vi "parse.issues.vi"(7 "series body":string, 8 "error in (no error)":errorcluster, 11 "ComicVine_class in":refnum<class "series_class.lvclass">) -> (0 "error out":errorcluster, 3 "ComicVine_class out":refnum<class "series_class.lvclass">)   [LabVIEW 2024, in "series_class.lvclass"]
uses:
  series_class.lvclass
  series_class.lvclass/series_class.ctl
  issue_class/issue_class.lvclass
  comic_class/comic_class.lvclass
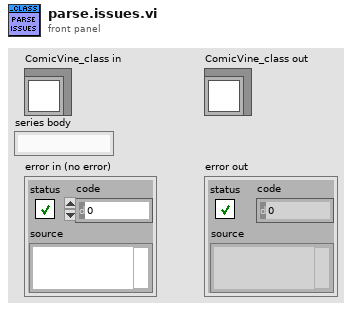
[diagram p1: front panel]
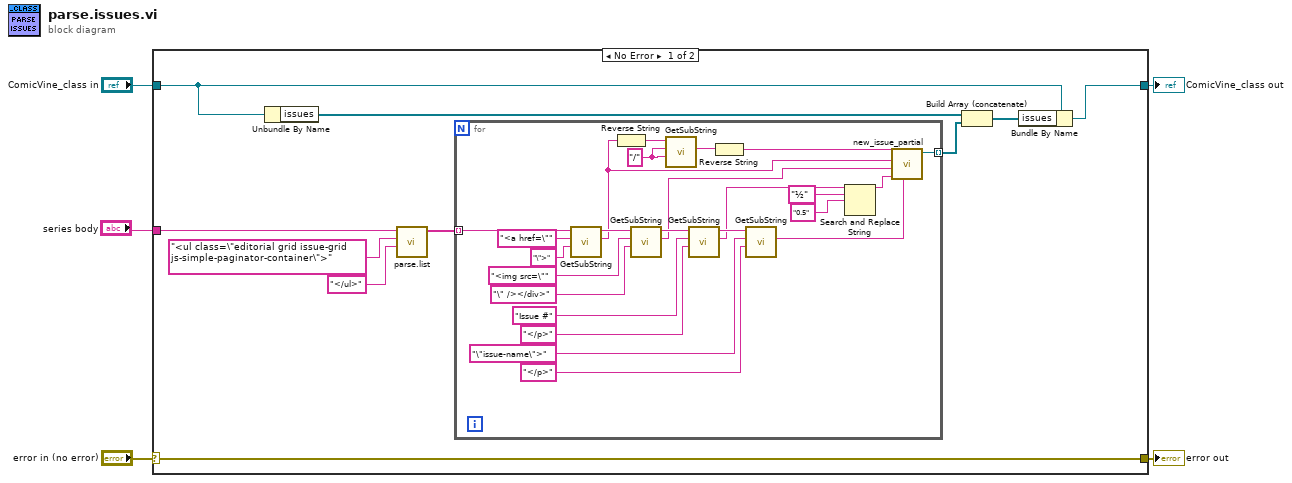
[diagram p0: block diagram]
diagram:
  n1 = case shown="No Error" "error in (no error)" {
    selector: "error in (no error)" -> [w15 w41]
    tunnel: [w15 w41] -> w4
    tunnel: [w11 w40] -> w2
    tunnel: "ComicVine_class in" -> [w13 w40]
    tunnel: "series body" -> [w9 _]
    frame No Error {
      n2 = Unbundle By Name(w13) -> ("issues"=w14:refnum<class "issue_class.lvclass">[])
      n3 = call "parse.list.vi"("div end"="</ul>", "div start"="<ul class=\"editorial grid issue-grid js-simple-paginator-container\">", "body"=w9) -> ("list array"=w6:string[])  [unwired: 8 in]
      n4 = for {
        tunnel: w6 -> [w39] mode=indexing
        tunnel: [w16] -> w10 mode=indexing
        w23 = "/" ("Start Search")
        n5 = call "GetSubString.vi"("End Search"="\">" ("Start Search"), "Start Search"="<a href=\"", "String In"=w39) -> ("Match"=w20:string, "Following String Out"=w36:string)  [unwired: 6 in, 1 out]
        n6 = Reverse String(1:w20) -> (0:w24:string)
        n7 = call "GetSubString.vi"("End Search"="\" /></div>" ("Start Search"), "Start Search"="<img src=\"", "String In"=w36) -> ("Match"=w19:string, "Following String Out"=w29:string)  [unwired: 6 in, 1 out]
        n8 = call "GetSubString.vi"("End Search"=w23, "Start Search"=w23, "String In"=w24) -> ("Match"=w22:string)  [unwired: 6 in, 2 out]
        n9 = call "GetSubString.vi"("End Search"="</p>" ("Start Search"), "Start Search"="Issue #", "String In"=w29) -> ("Match"=w25:string, "Following String Out"=w28:string)  [unwired: 6 in, 1 out]
        n10 = Reverse String(1:w22) -> (0:w21:string)
        n11 = call "GetSubString.vi"("End Search"="</p>" ("Start Search"), "Start Search"="\"issue-name\">", "String In"=w28) -> ("Match"=w17:string)  [unwired: 6 in, 2 out]
        n12 = Search and Replace String(input string=w25, search string="½" ("Start Search"), replace string="0.5" ("replace string (\"\")")) -> (result string=w18:string)  [unwired: 5 in, 3 out]
        n13 = call "new_issue_partial.vi"("name"=w17, "number"=w18, "small cover url"=w19, "url"=w20, "id"=w21) -> ("issue_class out"=w16:refnum<class "issue_class.lvclass">)  [unwired: 6 in]
      }
      n14 = Build Array (concatenate)(w14, w10) -> (w12:refnum<class "issue_class.lvclass">[])
      n15 = Bundle By Name(cluster=w13, "issues"=w12) -> (w11:refnum<class "series_class.lvclass">)
    }
    frame Error {
    }
  }
  "error out" <- w4
  "ComicVine_class out" <- w2
